vi "CLD 2  Elapsed Time Express Caller Self Solution.vi"() -> ()   [LabVIEW 2015]
doc: "CLD 2 Exercise"
panel:
  out "Time Has Elapsed":bool
  out "Elapsed Time (s)":dbl format="%#.2g"
  out "error out":errorcluster
  in  "Time Target (s)":dbl=4.0
  in  "Auto Reset (F)":bool=TRUE
  in  "error in (no error)":errorcluster
  in  "Timer Mode":enum16{"Reset", "Read Status", "Set Auto Reset"}(ring)
  in  "stop":bool
  # "Caller for the FGV"
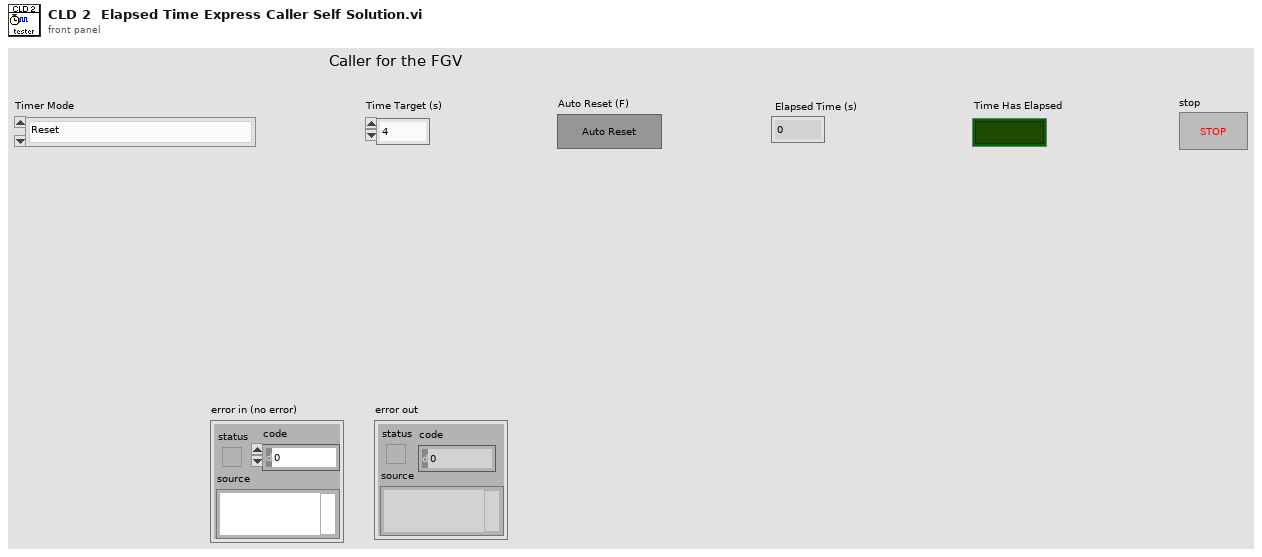
[diagram p1: front panel]
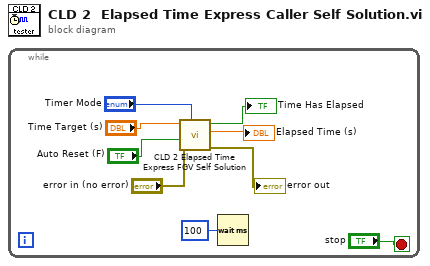
[diagram p0: block diagram]
diagram:
  n1 = while {
    stop <- "stop" stop-if-true
    n2 = call "CLD 2 Elapsed Time Express FGV Self Solution.vi"("Express Timer FGV Enum"="Timer Mode", "error in (no error)"="error in (no error)", "Auto Reset (F)"="Auto Reset (F)", "Time Target (s)"="Time Target (s)") -> ("error out"=→"error out":errorcluster, "Elapsed Time (s)"=→"Elapsed Time (s)":dbl, "Time Has Elapsed"=→"Time Has Elapsed":bool)  [unwired: 5 in]
    n3 = Wait (ms)(milliseconds to wait=u32 100) -> ()  [unwired: 1 out]
  }
